vi "senPID.vi"(1 "Numeric 3":dbl, 2 "Numeric 2":dbl, 3 "Numeric":dbl, 4 "String":string) -> (0 "String 2":string)   [LabVIEW 2017]
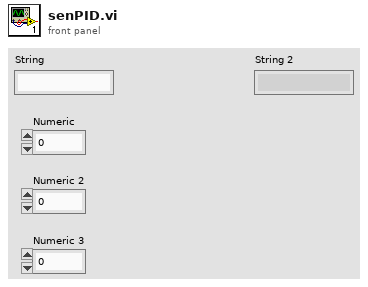
[diagram p1: front panel]
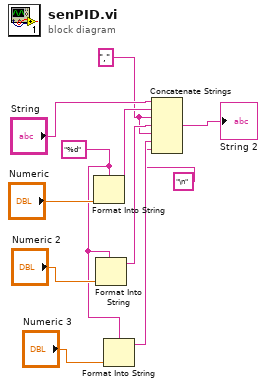
[diagram p0: block diagram]
diagram:
  w6 = ","
  w4 = "%d" ("format string")
  n1 = Format Into String(format string=w4, "Numeric") -> (resulting string=w9:string)  [unwired: 2 in, 1 out]
  n2 = Format Into String(format string=w4, "Numeric 2") -> (resulting string=w7:string)  [unwired: 2 in, 1 out]
  n3 = Format Into String(format string=w4, "Numeric 3") -> (resulting string=w3:string)  [unwired: 2 in, 1 out]
  n4 = Concatenate Strings("String", w9, w6, w7, w6, w3, "\n") -> (→"String 2":string)
